vi "Set Up Dialog - Conductivity.vi"() -> ()   [LabVIEW 2012]
panel:
  in  "Done":bool
  # "iWorx - Conductivity - Set Up"
  # "Calibration Instructions"
  # "1. Connect the IX-MYDAQ Sensor Adaptor to the NI myDAQ.\n\n2. Connect the CMN-100 Conductivity Sensor to the IX-MYDAQ.\n\n3. Connect the NI myDAQ to your computer using a USB cable.\n\n4. The CMN-100 should be calibrated within the expected range. \n\nFor example: If the expected range is 500uS to 1000uS perform a 2 point calibration with the first point (SP1) at 400uS and the second point (SP2) at 1000uS."
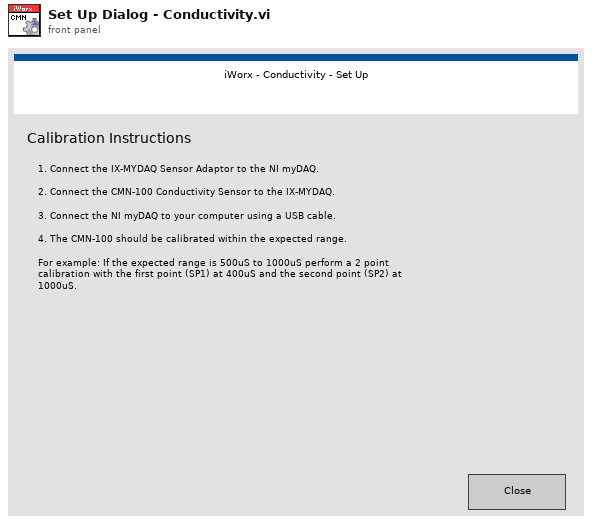
[diagram p1: front panel]
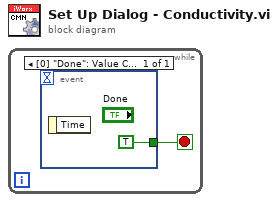
[diagram p0: block diagram]
diagram:
  n1 = while {
    stop <- w1 stop-if-true
    n2 = event shown="[0] \"Done\": Value Change;  Panel Close" {
      selector: _ -> [_]
      dyn-events: _ -> [_]
      timeout: _ -> [_]
      tunnel: [TRUE] -> w1
      event "Done": Value Change; Panel Close {
        n3 = event-data() -> ()  [unwired: 1 in, 1 out]
      }
    }
  }
